vi "Panel Update Dryer Details.vi"(0 "Dryer Details In":T1 {"Stop Dryer" items=["NO", "YES"]; "24 Hour Water Injection" items=["NO", "YES"]; "Run w/o Newfi" items=["NO", "YES"]}) -> (4 "Dryer Details Out":T1 {"Stop Dryer" items=["NO", "YES"]; "24 Hour Water Injection" items=["NO", "YES"]; "Run w/o Newfi" items=["NO", "YES"]}, 6 "New Filenames":bool, 8 "Updated":bool)   [LabVIEW 2012]
uses:
  Dryer Details.ctl
panel:
  in  "Tab Control":enum32{"Update Panel", "Debug"}(tab)
  in  "Stop Dryer":i32(ring) items=["NO", "YES"]
  in  "24 Hour Water Injection":i32(ring) items=["NO", "YES"]
  in  "Run w/o Newfi":i32(ring) items=["NO", "YES"]
  out "Station":string
  in  "Lab ID":string
  in  "Notes":string
  in  "TR Number":string
  in  "stop":bool
  in  "Cycle Count Day":string
  in  "Cycle Count Night":string
  in  "Time On Day":string
  in  "Time On Night":string
  in  "Cancel":bool
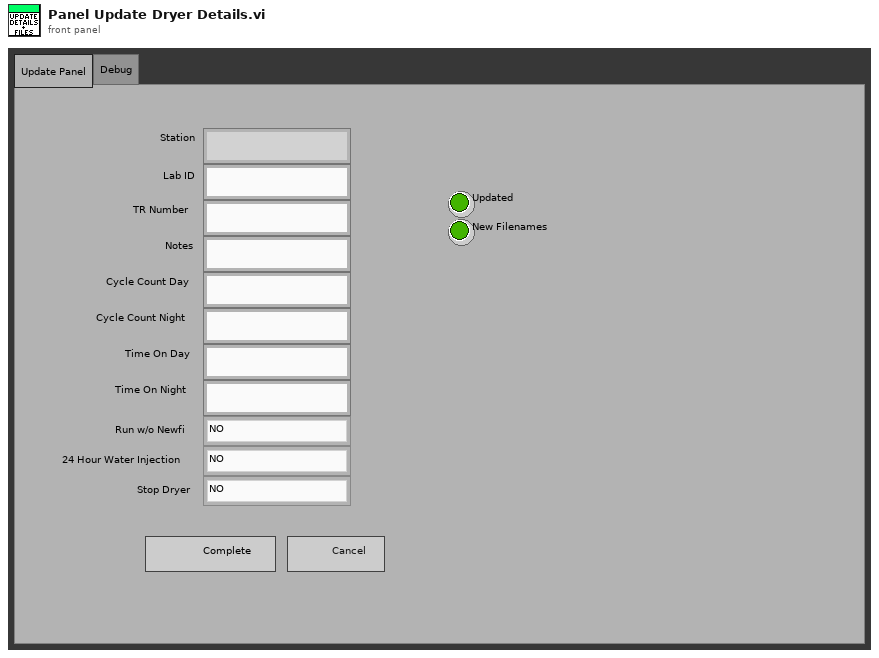
[diagram p1: front panel]
types:
  T1 = typedef "Dryer Details.ctl" = cluster{"Station":string, "Cycle Count Day":string, "Status":string, "Debug ASCII":string, "Notes":string, "Lab ID":string, "Total Time On":string, "TR Number":string, "Cycle Count Night":string, "Time On Day":string, "Time On Night":string, "Run w/o Newfi":i32, "24 Hour Water Injection":i32, "Stop Dryer":i32}
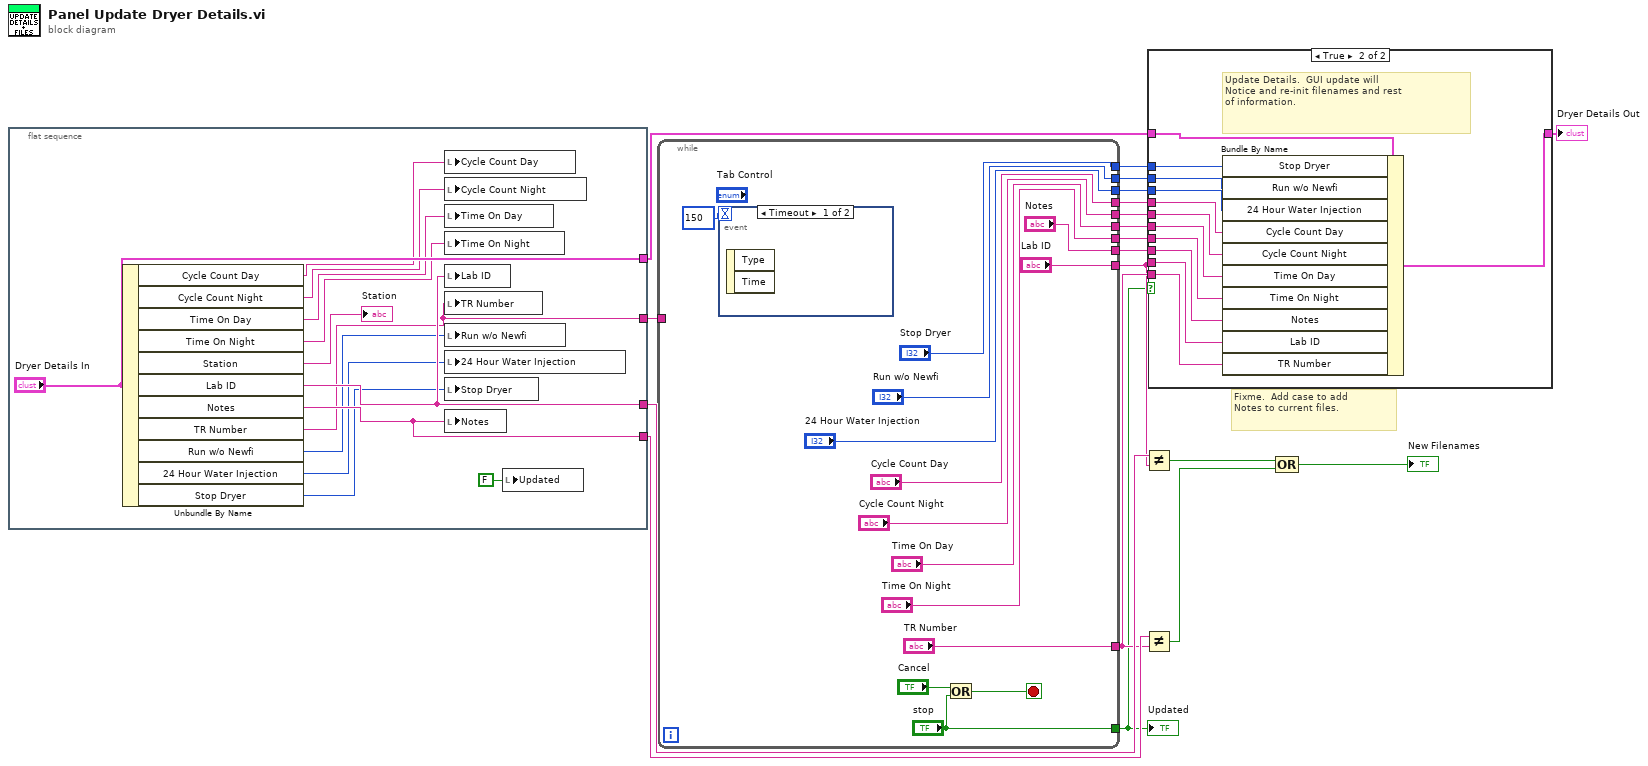
[diagram p0: block diagram]
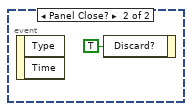
[diagram p3: hidden frame]
diagram:
  # "Fixme.  Add case to add\nNotes to current files."
  n1 = flat-sequence {
    tunnel: [w29] -> w19
    tunnel: [w31] -> w16
    tunnel: [w30] -> w15
    tunnel: ["Dryer Details In"] -> w10
    frame #0 {
      n2 = Unbundle By Name("Dryer Details In") -> ("Cycle Count Day"=w24:string, "Cycle Count Night"=w25:string, "Time On Day"=w26:string, "Time On Night"=w27:string, "Station"=→"Station":string, "Lab ID"=w31:string, "Notes"=w30:string, "TR Number"=w29:string, "Run w/o Newfi"=w22:i32, "24 Hour Water Injection"=w23:i32, "Stop Dryer"=w21:i32)
      n3 = local write "Cycle Count Day"(w24) -> ()
      n4 = local write "Cycle Count Night"(w25) -> ()
      n5 = local write "Time On Day"(w26) -> ()
      n6 = local write "Time On Night"(w27) -> ()
      n7 = local write "Lab ID"(w31) -> ()
      n8 = local write "TR Number"(w29) -> ()
      n9 = local write "Run w/o Newfi"(w22) -> ()
      n10 = local write "24 Hour Water Injection"(w23) -> ()
      n11 = local write "Stop Dryer"(w21) -> ()
      n12 = local write "Notes"(w30) -> ()
      n13 = local write "Updated"(FALSE ("Updated")) -> ()
    }
  }
  n14 = while {
    tunnel: w19 -> [_]
    tunnel: ["Lab ID"] -> w12
    tunnel: ["TR Number"] -> w13
    tunnel: ["Notes"] -> w11
    tunnel: ["Time On Night"] -> w8
    tunnel: ["Time On Day"] -> w7
    tunnel: ["Cycle Count Night"] -> w6
    tunnel: ["Cycle Count Day"] -> w5
    tunnel: ["stop"] -> w4
    tunnel: ["Run w/o Newfi"] -> w3
    tunnel: ["24 Hour Water Injection"] -> w2
    tunnel: ["Stop Dryer"] -> w1
    stop <- w38 stop-if-true
    n15 = event shown="[0] Timeout" {
      selector: _ -> [_ _]
      dyn-events: _ -> [_ _]
      timeout: 150 ("milliseconds to wait") -> [_ _]
      event Timeout {
        n16 = event-data() -> ()  [unwired: 1 in, 2 out]
      }
      event Panel Close? {
        n17 = event-data() -> ()  [unwired: 1 in, 2 out]
        n18 = event-data("Discard?"=TRUE) -> ()  [unwired: 1 in, 1 out]
      }
    }
    n19 = Or(x="Cancel", y="stop") -> (x .or. y?=w38:bool)
  }
  "Updated" <- w4
  n20 = Not Equal?(x=w16, y=w12) -> (x != y?=w18:bool)
  n21 = Not Equal?(x=w15, y=w13) -> (x != y?=w17:bool)
  n22 = case shown="True" w4 {
    tunnel: w13 -> [_ w57]
    tunnel: w12 -> [_ w56]
    tunnel: w11 -> [_ w59]
    tunnel: w10 -> [w48 w60]
    tunnel: [w48 w58] -> w9
    tunnel: w8 -> [_ w55]
    tunnel: w7 -> [_ w54]
    tunnel: w6 -> [_ w53]
    tunnel: w5 -> [_ w52]
    tunnel: w3 -> [_ w51]
    tunnel: w2 -> [_ w50]
    tunnel: w1 -> [_ w49]
    frame False {
    }
    frame True {
      # "Update Details.  GUI update will\nNotice and re-init filenames and rest\nof information."
      n23 = Bundle By Name(cluster=w60, "Stop Dryer"=w49, "Run w/o Newfi"=w51, "24 Hour Water Injection"=w50, "Cycle Count Day"=w52, "Cycle Count Night"=w53, "Time On Day"=w54, "Time On Night"=w55, "Notes"=w59, "Lab ID"=w56, "TR Number"=w57) -> (w58:T1)
    }
  }
  "Dryer Details Out" <- w9
  n24 = Compound Arithmetic op=OR(w18, w17) -> (→"New Filenames":bool)
